vi "Init.vi"(8 "error in (no error)":errorcluster, 11 "MENSAJES in":refnum<class "MENSAJES.lvclass">) -> (0 "error out":errorcluster, 3 "MENSAJES out":refnum<class "MENSAJES.lvclass">)   [LabVIEW 2019, in "MENSAJES.lvlib" / "MENSAJES.lvclass"]
uses:
  MENSAJES.lvclass
  MENSAJES.lvclass/MENSAJES.ctl
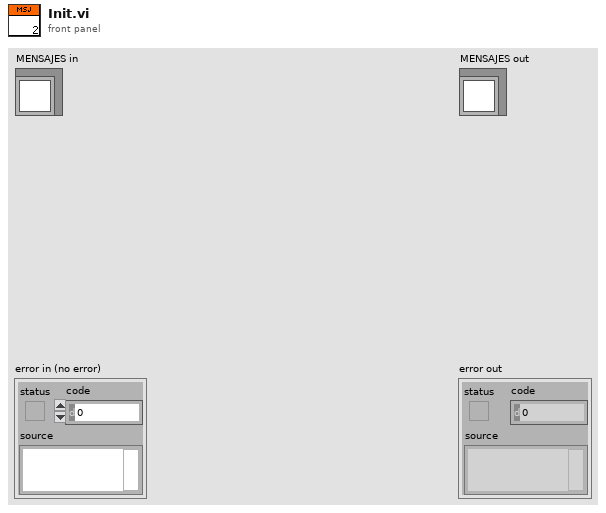
[diagram p1: front panel]
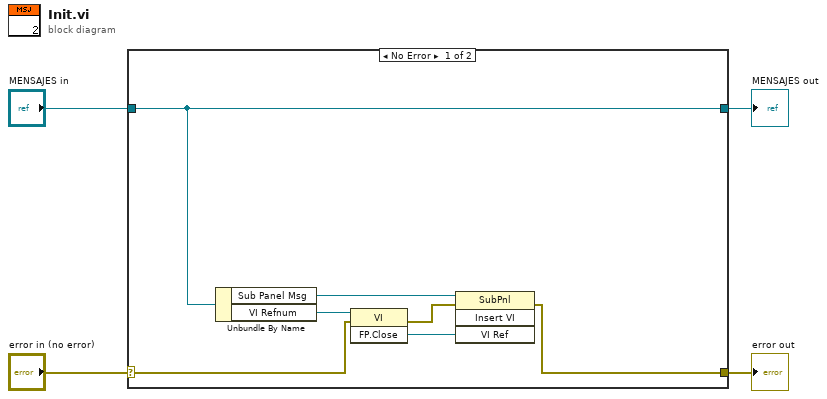
[diagram p0: block diagram]
diagram:
  n1 = case shown="No Error" "error in (no error)" {
    selector: "error in (no error)" -> [w8 w13]
    tunnel: [w7 w13] -> w2
    tunnel: [w6 w12] -> w1
    tunnel: "MENSAJES in" -> [w6 w12]
    frame No Error {
      n2 = Unbundle By Name(w6) -> ("Sub Panel Msg"=w5:refnum<vi>, "VI Refnum"=w11:refnum<vi>)
      n3 = invoke class="VI" method="FP.Close"(reference=w11, error in=w8) -> (reference out=w10:refnum<vi>, error out=w9:errorcluster)  [unwired: 1 in, 1 out]
      n4 = invoke class="SubPnl" method="Insert VI"(reference=w5, error in=w9, "VI Ref"=w10) -> (error out=w7:errorcluster)  [unwired: 1 in, 3 out]
    }
    frame Error {
    }
  }
  "error out" <- w2
  "MENSAJES out" <- w1
